vi "Config AM Modulation.vi"(0 "VISA Resource Name":refnum<visa-resource-name>, 1 "Path (0:1)":enum16{"1", "2", "WIDE BAND"}(ring), 2 "Status (T:ON)":bool=TRUE, 3 "EXT Source Coupling (F:DC)":bool, 4 "AM Depth Couple (F:OFF)":bool, 5 "error in (no error)":errorcluster {"code" format="%.0x"}, 6 "AM Depth (0.1)":dbl=0.1 format="%.1f", 7 "Dual/Swept Parameters":T1={"Alt Frequency (400.0)"=400.0, "Alt Freq Amplitude (50.0)"=50.0, "Sweep Time (100.0)"=100.0, "Sweep Trigger (0:IMMEDIATE)"=enum."IMMEDIATE"} {"Sweep Time (100.0)" format="%.1f"; "Alt Freq Amplitude (50.0)" format="%.1f"; "Alt Frequency (400.0)" format="%.1f"}, 8 "AM Source (0:Internal)":enum16{"INTERNAL", "EXT1", "EXT2"}(ring), 10 "AM Rate (400.0)":dbl=400.0 format="%.1f", 12 "AM Waveform (0:SINE)":T2(ring)) -> (14 "VISA Resource Name Out":refnum<visa-resource-name>, 19 "error out":errorcluster {"code" format="%.0x"})   [LabVIEW 2014, in "Agilent ESG Series.lvlib"]
doc: "This VI is used to set the modulation controls and the parameters associated with amplitude modulated signals."
uses:
  Agilent ESG Series.lvlib
panel:
  # "ON"
  # "OFF"
  # "AC"
  # "DC"
  # "ON"
  # "OFF"
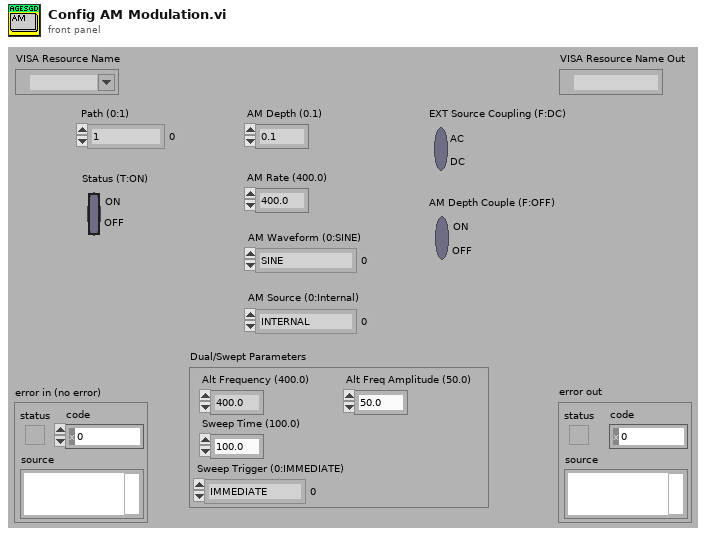
[diagram p1: front panel]
types:
  T1 = cluster{"Alt Frequency (400.0)":dbl, "Alt Freq Amplitude (50.0)":dbl, "Sweep Time (100.0)":dbl, "Sweep Trigger (0:IMMEDIATE)":enum16{"IMMEDIATE", "BUS", "EXTERNAL", "KEY"}}
  T2 = enum16{"SINE", "TRIANGLE", "SQUARE", "RAMP", "NOISE", "DUAL SINE", "SWEPT SINE"}
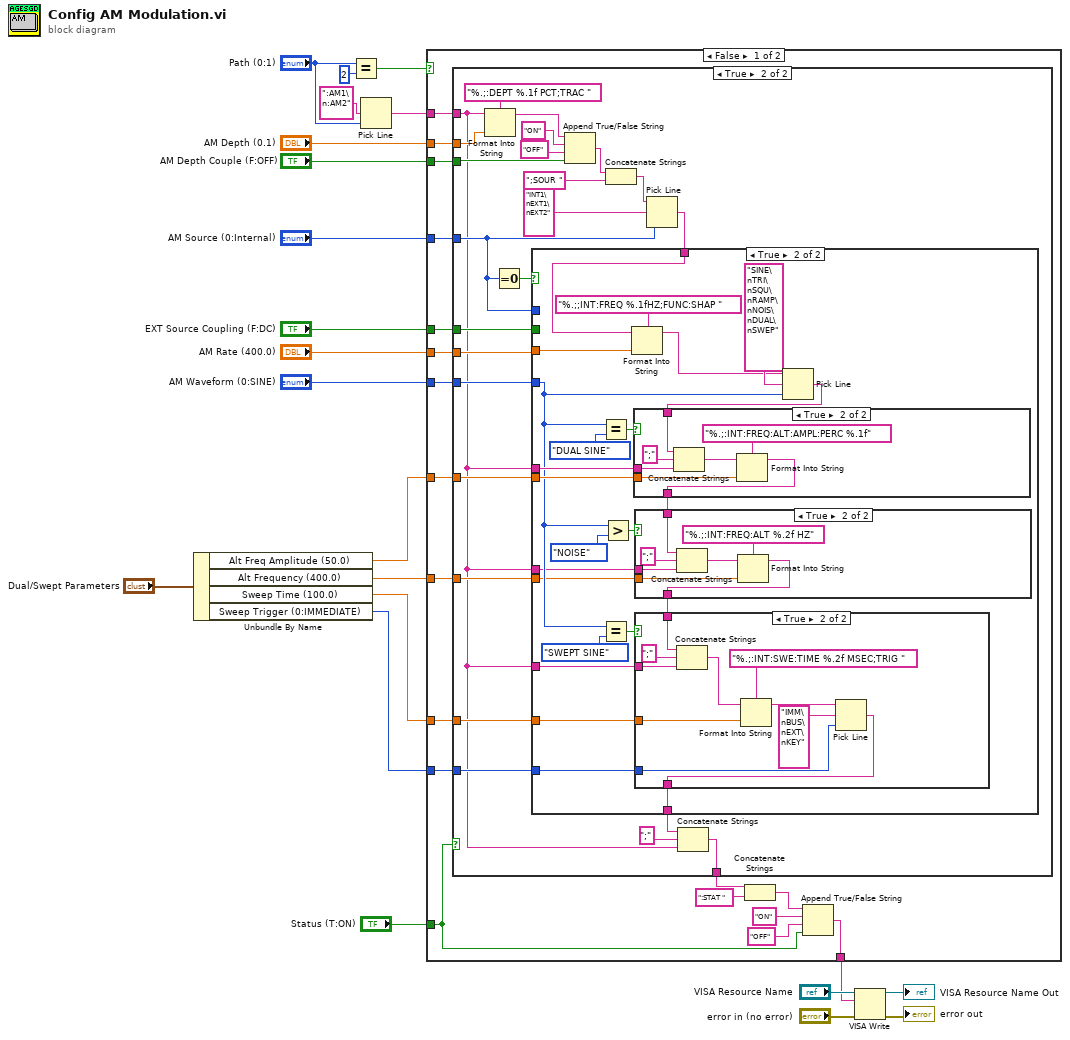
[diagram p0: block diagram]
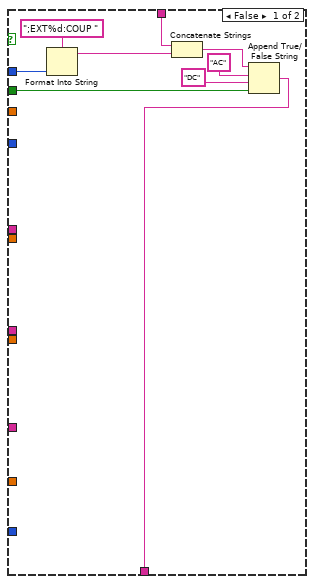
[diagram p3: hidden frame]
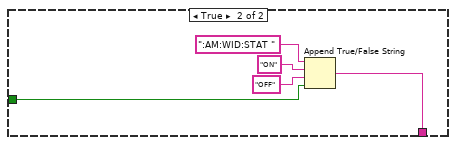
[diagram p7: hidden frame]
diagram:
  n1 = Unbundle By Name("Dual/Swept Parameters") -> ("Alt Freq Amplitude (50.0)"=w4:dbl, "Alt Frequency (400.0)"=w3:dbl, "Sweep Time (100.0)"=w2:dbl, "Sweep Trigger (0:IMMEDIATE)"=w1:enum16{"IMMEDIATE", "BUS", "EXTERNAL", "KEY"})
  n2 = Equal?(x="Path (0:1)", y=i8 2) -> (x = y?=w19:bool)
  n3 = Pick Line(multi-line string=":AM1\n:AM2" ("true string"), line index="Path (0:1)") -> (output string=w10:string)  [unwired: 1 in]
  n4 = case shown="False" w19 {
    tunnel: "AM Depth (0.1)" -> [w40 _]
    tunnel: "AM Depth Couple (F:OFF)" -> [w39 _]
    tunnel: "AM Source (0:Internal)" -> [w38 _]
    tunnel: [w33 w125] -> w13
    tunnel: w10 -> [w31 _]
    tunnel: "Status (T:ON)" -> [w23 w126]
    tunnel: "EXT Source Coupling (F:DC)" -> [w30 _]
    tunnel: "AM Rate (400.0)" -> [w29 _]
    tunnel: "AM Waveform (0:SINE)" -> [w28 _]
    tunnel: w4 -> [w27 _]
    tunnel: w3 -> [w26 _]
    tunnel: w2 -> [w25 _]
    tunnel: w1 -> [w24 _]
    frame False {
      n5 = case shown="True" w23 {
        tunnel: w24 -> [_ w65]
        tunnel: w25 -> [_ w64]
        tunnel: w26 -> [_ w63]
        tunnel: w27 -> [_ w62]
        tunnel: w28 -> [_ w61]
        tunnel: w29 -> [_ w60]
        tunnel: w30 -> [_ w59]
        tunnel: w31 -> [w41 w43]
        tunnel: [w41 w42] -> w32
        tunnel: w38 -> [_ w46]
        tunnel: w39 -> [_ w45]
        tunnel: w40 -> [_ w44]
        frame False {
        }
        frame True {
          n6 = Format Into String(format string="%.;:DEPT %.1f PCT;TRAC ", initial string=w43, w44) -> (resulting string=w52:string)  [unwired: 1 in, 1 out]
          n7 = Equal To 0?(x=w46) -> (x = 0?=w57:bool)
          n8 = Append True/False String(1:w45, 2:"OFF" ("false string"), 3:"ON" ("true string"), 4:w52) -> (0:w53:string)
          n9 = Concatenate Strings(w53, ";SOUR ") -> (w55:string)
          n10 = Pick Line(string ("")=w55, multi-line string="INT1\nEXT1\nEXT2", line index=w46) -> (output string=w58:string)
          n11 = case shown="True" w57 {
            tunnel: w58 -> [w73 w97]
            tunnel: [w70 w86] -> w48
            tunnel: w46 -> [w69 _]
            tunnel: w59 -> [w66 _]
            tunnel: w60 -> [_ w96]
            tunnel: w61 -> [_ w80]
            tunnel: w62 -> [_ w89]
            tunnel: w63 -> [_ w79]
            tunnel: w65 -> [_ w84]
            tunnel: w64 -> [_ w85]
            tunnel: w43 -> [_ w83]
            tunnel: w43 -> [_ w82]
            tunnel: w43 -> [_ w78]
            frame False {
              n12 = Format Into String(format string=";EXT%d:COUP ", w69) -> (resulting string=w67:string)  [unwired: 2 in, 1 out]
              n13 = Concatenate Strings(w73, w67) -> (w72:string)
              n14 = Append True/False String(1:w66, 2:"DC" ("false string"), 3:"AC" ("true string"), 4:w72) -> (0:w70:string)
            }
            frame True {
              n15 = Equal?(x=w80, y=T2."DUAL SINE") -> (x = y?=w91:bool)
              n16 = Equal?(x=w80, y=T2."SWEPT SINE") -> (x = y?=w87:bool)
              n17 = Greater?(x=w80, y=T2."NOISE") -> (0:w75:bool)
              n18 = Format Into String(format string="%.;;INT:FREQ %.1fHZ;FUNC:SHAP ", initial string=w97, w96) -> (resulting string=w93:string)  [unwired: 1 in, 1 out]
              n19 = Pick Line(string ("")=w93, multi-line string="SINE\nTRI\nSQU\nRAMP\nNOIS\nDUAL\nSWEP", line index=w80) -> (output string=w90:string)
              n20 = case shown="True" w91 {
                tunnel: w90 -> [w117 w119]
                tunnel: [w117 w118] -> w76
                tunnel: w89 -> [_ w123]
                tunnel: w83 -> [_ w120]
                frame False {
                }
                frame True {
                  n21 = Concatenate Strings(w119, ";" ("true string"), w120) -> (w122:string)
                  n22 = Format Into String(format string="%.;:INT:FREQ:ALT:AMPL:PERC %.1f", initial string=w122, w123) -> (resulting string=w118:string)  [unwired: 1 in, 1 out]
                }
              }
              n23 = case shown="True" w75 {
                tunnel: w76 -> [w98 w100]
                tunnel: [w98 w99] -> w77
                tunnel: w79 -> [_ w104]
                tunnel: w78 -> [_ w101]
                frame False {
                }
                frame True {
                  n24 = Concatenate Strings(w100, ";" ("true string"), w101) -> (w103:string)
                  n25 = Format Into String(format string="%.;:INT:FREQ:ALT %.2f HZ", initial string=w103, w104) -> (resulting string=w99:string)  [unwired: 1 in, 1 out]
                }
              }
              n26 = case shown="True" w87 {
                tunnel: w77 -> [w106 w107]
                tunnel: [w106 w113] -> w86
                tunnel: w85 -> [_ w112]
                tunnel: w84 -> [_ w111]
                tunnel: w82 -> [_ w109]
                frame False {
                }
                frame True {
                  n27 = Concatenate Strings(w107, ";" ("true string"), w109) -> (w108:string)
                  n28 = Format Into String(format string="%.;:INT:SWE:TIME %.2f MSEC;TRIG ", initial string=w108, w112) -> (resulting string=w116:string)  [unwired: 1 in, 1 out]
                  n29 = Pick Line(string ("")=w116, multi-line string="IMM\nBUS\nEXT\nKEY", line index=w111) -> (output string=w113:string)
                }
              }
            }
          }
          n30 = Concatenate Strings(w48, ";" ("true string"), w43) -> (w42:string)
        }
      }
      n31 = Concatenate Strings(w32, ":STAT ") -> (w35:string)
      n32 = Append True/False String(1:w23, 2:"OFF" ("false string"), 3:"ON" ("true string"), 4:w35) -> (0:w33:string)
    }
    frame True {
      n33 = Append True/False String(1:w126, 2:"OFF" ("false string"), 3:"ON" ("true string"), 4:":AM:WID:STAT ") -> (0:w125:string)
    }
  }
  n34 = VISA Write(VISA resource name="VISA Resource Name", write buffer=w13, error in (no error)="error in (no error)") -> (VISA resource name out=→"VISA Resource Name Out":refnum<visa-resource-name>, error out=→"error out":errorcluster)  [unwired: 1 out]
